vi "Handle Error.vi"(8 "error in (no error)":errorcluster, 11 "Mercury Temperature Controller in":refnum<class "Mercury Temperature Controller.lvclass">) -> (0 "error out":errorcluster, 2 "stop actor?":bool=TRUE, 3 "Mercury Temperature Controller out":refnum<class "Mercury Temperature Controller.lvclass">)   [LabVIEW 2015, in "Mercury Temperature Controller.lvclass"]
doc: "(<B>Filename</B>: Actor Framework.lvlib:Actor.lvclass:Handle Error.vi)\n\nDefines how the actor handles an error that occurred while processing a message. By default, this method does nothing except stop the actor."
uses:
  Temperature Controller/Mercury Temperature Controller.lvclass
  <vilib>/ActorFramework/Actor/Actor.lvclass
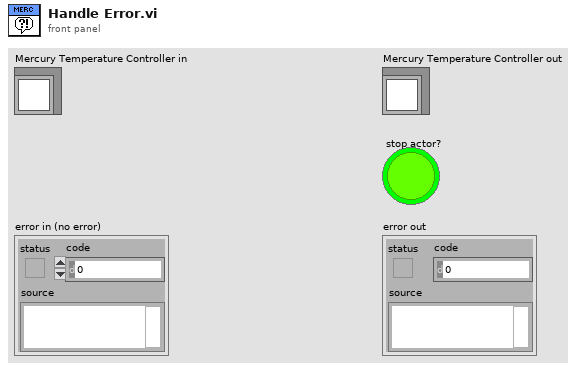
[diagram p1: front panel]
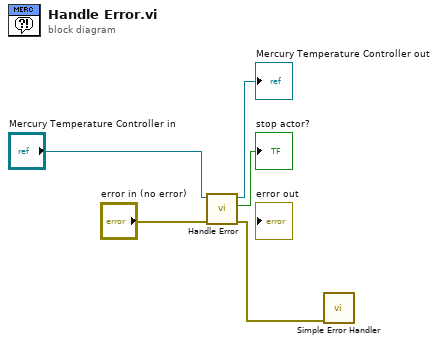
[diagram p0: block diagram]
diagram:
  n1 = call-parent "Handle Error.vi"("error in (no error)"="error in (no error)", "Actor in"="Mercury Temperature Controller in") -> ("error out"=w1:errorcluster, "stop actor?"=→"stop actor?":bool, "Actor out"=→"Mercury Temperature Controller out":refnum<class "Mercury Temperature Controller.lvclass">)  [unwired: 7 in]
  n2 = call <vilib>:"Simple Error Handler.vi"("error in (no error)"=w1) -> ()  [unwired: 4 in, 5 out]
